vi "GyroOpen.vi"(8 "refnum name":string="My I2C RefNum", 9 "Device Address":u8, 10 "Controller":T1, 11 "I2C Bus":T2=enum."Invalid") -> ()   [LabVIEW 2014]
uses:
  <vilib>/Rock Robotics/SystemInterfaces/i2clib/i2c_bus.ctl
  <vilib>/Rock Robotics/SystemInterfaces/Typedef/FPGA_TypedefDigitalModule.ctl
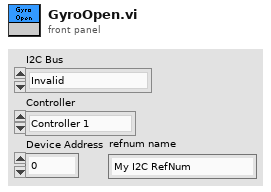
[diagram p1: front panel]
types:
  T1 = typedef "FPGA_TypedefDigitalModule.ctl" = enum16{"Controller 1"}
  T2 = typedef "i2c_bus.ctl" = enum16{"I2C On-Board", "I2C MXP", "Invalid"}
  T3 = typedef "WPI_I2CDevRef.ctl" = cluster{"DevStatus":errorcluster, "Controller":T1, "Device Address":u8, "Handle":i32, "I2C Bus":T2}
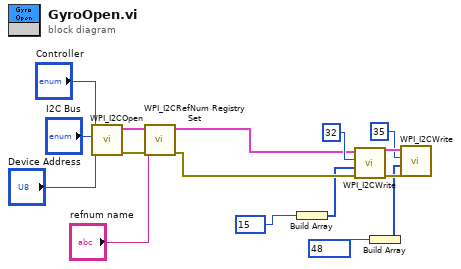
[diagram p0: block diagram]
diagram:
  n1 = call <vilib>:"WPI_I2COpen.vi"("Device Address"="Device Address", "I2C Bus"="I2C Bus", "Controller"="Controller") -> ("error out"=w16:errorcluster, "I2CDevRef"=w15:T3)  [unwired: 7 in]
  n2 = call <vilib>:"WPI_I2CRefNum Registry Set.vi"("error in (no error)"=w16, "refnum name"="refnum name", "I2CDevRef"=w15) -> ("error out"=w3:errorcluster, "I2CDevRef"=w4:T3)  [unwired: 7 in]
  n3 = Build Array(u8 15) -> (w1:u8[])
  n4 = call <vilib>:"WPI_I2CWrite.vi"("error in (no error)"=w3, "I2CDataToSend"=w1, "I2CRegister"=u8 32, "I2CDevRef"=w4) -> ("error out"=w8:errorcluster, "I2CDevRef"=w9:T3)  [unwired: 6 in]
  n5 = Build Array(u8 48) -> (w5:u8[])
  n6 = call <vilib>:"WPI_I2CWrite.vi"("error in (no error)"=w8, "I2CDataToSend"=w5, "I2CRegister"=u8 35, "I2CDevRef"=w9) -> ()  [unwired: 6 in, 2 out]
